vi "CRYBackup All.vi"(11 "sOption":string) -> ()   [LabVIEW 2013]
uses:
  CRYSystem/Typedef Control/CRYData Cluster Array.ctl
  CRYSystem/Typedef Control/CRYData Cluster.ctl
  CRYSystem/Typedef Control/CRYResult Cluster Array.ctl
  CRYSystem/Typedef Control/CRYResult Cluster.ctl
  CRYSystem/Typedef Control/CRYWaveform Cluster Array.ctl
  CRYSystem/Typedef Control/CRYWaveform Cluster.ctl
  CRYProject/CRYProject Editor Global.vi
  Global/CRYCurves Array Global.vi
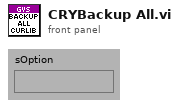
[diagram p1: front panel]
types:
  T1 = typedef "CRYWaveform Cluster Array.ctl" = T2[]
  T2 = typedef "CRYWaveform Cluster.ctl" = cluster{"Waveform":cluster{"X0":dbl, "dX":dbl, "Y":sgl[]}, "X data":u16, "Y data":u16, "Y axis":u16, "X unit":string, "Y unit":string, "Y dB ref":dbl, "display Y":bool, "display X":bool, "Overload?":bool, "Test Info":string, "Step No.":i32, "Name":string, "protected":bool, "Sqc history":string[], "Signal Channel ID":i32, "Plot Settings":cluster{"Color":u32, "Interpolation":u8, "Point Style":u8, "Line Style":u8, "Point Color":u32, "Line Width":u8, "Bar Plot Style":u8, "Fill To":i16}, "AutoProtect":bool}
  T3 = typedef "CRYResult Cluster Array.ctl" = T4[]
  T4 = typedef "CRYResult Cluster.ctl" = cluster{"Name":string, "Margin":dbl, "unit":string, "Verdict":bool, "Limit":string, "Max/Min":string, "protected":bool, "Step No.":i32, "Test Info":string, "AutoProtect":bool}
  T5 = typedef "CRYData Cluster.ctl" = cluster{"Name":string, "Curve":cluster{"x":dbl, "y":dbl, "z":dbl}[], "X data":u16, "Y data":u16, "Z data":u16, "X axis":u16, "Y axis":u16, "Z axis":u16, "X unit":string, "Y unit":string, "Z unit":string, "X dB ref":dbl, "Y dB ref":dbl, "Z dB ref":dbl, "single val":bool, "protected":bool, "display X":bool, "display Y":bool, "display Z":bool, "Test Info":string, "Step No.":i32, "Plot Settings":cluster{"Color":u32, "Interpolation":u8, "Point Style":u8, "Line Style":u8, "Point Color":u32, "Line Width":u8, "Bar Plot Style":u8, "Fill To":i16}, "AutoProtect":bool}
  T6 = typedef "CRYData Cluster Array.ctl" = T5[]
  T7 = typedef "CRYStep.ctl" = cluster{"No.VI":i32, "Category":string, "StepName":string, "Seq setup flattened":string, "Comment":string, "Steps config.":bool[], "Jump config":i32[], "Start":dbl, "Increment":dbl, "Name":string, "Unit":string, "Y data":u16, "Y prefix":string, "Y dB ref":dbl, "Y unit":string, "Repeat State Array":cluster{"Start":dbl, "Increment":dbl, "Count":i32, "Num":i32}[]}
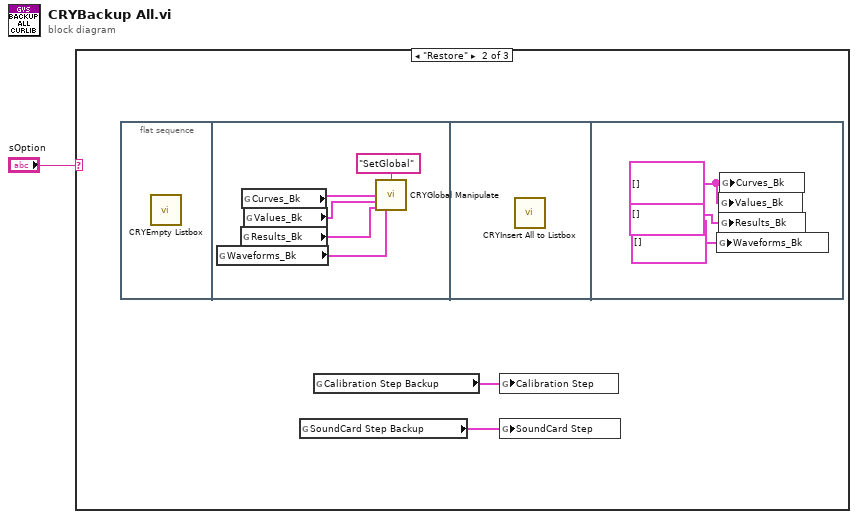
[diagram p0: block diagram]
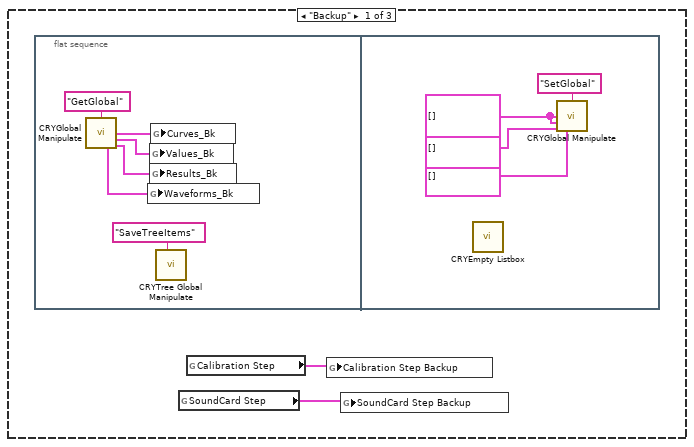
[diagram p2: hidden frame]
diagram:
  n1 = case shown="\"Restore\"" "sOption" {
    frame "Backup" {
      n2 = flat-sequence {
        frame #0 {
          n3 = call "CRYGlobal Manipulate.vi"("sAction"="GetGlobal") -> ("Curves Out"=w8:T5[], "Values Out"=w7:T5[], "WFM Out"=w5:T2[], "Results Out"=w6:T4[])  [unwired: 8 in, 3 out]
          n4 = global write "CRYCurves Array Global.vi" "Waveforms_Bk"(w5) -> ()
          n5 = global write "CRYCurves Array Global.vi" "Values_Bk"(w7) -> ()
          n6 = global write "CRYCurves Array Global.vi" "Results_Bk"(w6) -> ()
          n7 = global write "CRYCurves Array Global.vi" "Curves_Bk"(w8) -> ()
          n8 = call "CRYTree Global Manipulate.vi"("sAction"="SaveTreeItems") -> ()  [unwired: 7 in, 4 out]
        }
        frame #1 {
          w12 = T6 [] ("Curve&Value array")
          n9 = call "CRYEmpty Listbox.vi"() -> ()  [unwired: 1 out]
          n10 = call "CRYGlobal Manipulate.vi"("sAction"="SetGlobal", "Curves"=w12, "Values"=w12, "Results"=T3 [] ("Result array"), "WFM"=T1 [] ("Waveform Array")) -> ()  [unwired: 4 in, 7 out]
        }
      }
      n11 = global read "CRYProject Editor Global.vi" "SoundCard Step"() -> (w2:T7)
      n12 = global read "CRYProject Editor Global.vi" "Calibration Step"() -> (w3:T7)
      n13 = global write "CRYProject Editor Global.vi" "Calibration Step Backup"(w3) -> ()
      n14 = global write "CRYProject Editor Global.vi" "SoundCard Step Backup"(w2) -> ()
    }
    frame "Restore" {
      n15 = flat-sequence {
        frame #0 {
          n16 = call "CRYEmpty Listbox.vi"() -> ()  [unwired: 1 out]
        }
        frame #1 {
          n17 = global read "CRYCurves Array Global.vi" "Waveforms_Bk"() -> (w16:T1)
          n18 = global read "CRYCurves Array Global.vi" "Results_Bk"() -> (w17:T3)
          n19 = global read "CRYCurves Array Global.vi" "Curves_Bk"() -> (w19:T6)
          n20 = global read "CRYCurves Array Global.vi" "Values_Bk"() -> (w18:T6)
          n21 = call "CRYGlobal Manipulate.vi"("sAction"="SetGlobal", "Curves"=w19, "Values"=w18, "Results"=w17, "WFM"=w16) -> ()  [unwired: 4 in, 7 out]
        }
        frame #2 {
          n22 = call "CRYInsert All to Listbox.vi"() -> ()  [unwired: 1 in, 11 out]
        }
        frame #3 {
          w23 = T6 [] ("Curve&Value array")
          n23 = global write "CRYCurves Array Global.vi" "Waveforms_Bk"(T1 [] ("Waveform Array")) -> ()
          n24 = global write "CRYCurves Array Global.vi" "Values_Bk"(w23) -> ()
          n25 = global write "CRYCurves Array Global.vi" "Results_Bk"(T3 [] ("Result array")) -> ()
          n26 = global write "CRYCurves Array Global.vi" "Curves_Bk"(w23) -> ()
        }
      }
      n27 = global read "CRYProject Editor Global.vi" "SoundCard Step Backup"() -> (w14:T7)
      n28 = global read "CRYProject Editor Global.vi" "Calibration Step Backup"() -> (w15:T7)
      n29 = global write "CRYProject Editor Global.vi" "Calibration Step"(w15) -> ()
      n30 = global write "CRYProject Editor Global.vi" "SoundCard Step"(w14) -> ()
    }
    frame Default {
    }
  }
